vi "Read State DVR.vi"(8 "error in (no error)":errorcluster, 11 "Check Ozone Stability in":refnum<class "Check Ozone Stability.lvclass">) -> (0 "error out":errorcluster, 2 "State DVR":refnum<data-value>, 3 "Check Ozone Stability out":refnum<class "Check Ozone Stability.lvclass">)   [LabVIEW 2013, in "Check Ozone Stability.lvclass"]
uses:
  Check Ozone Stability.lvclass
  Data/cPAS Data.lvclass
  Check Ozone Stability.lvclass/Check Ozone Stability.ctl
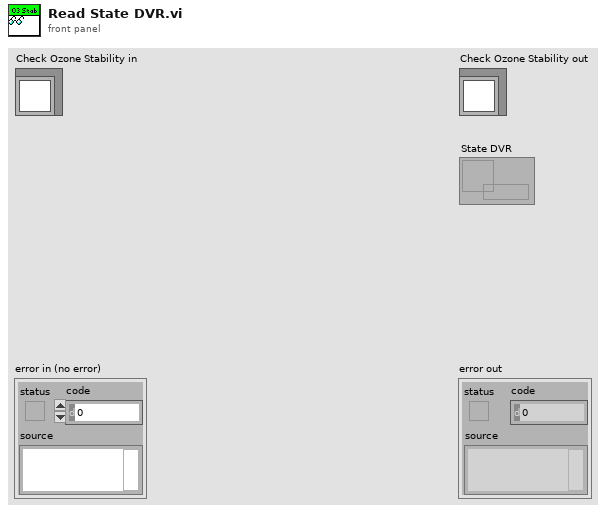
[diagram p1: front panel]
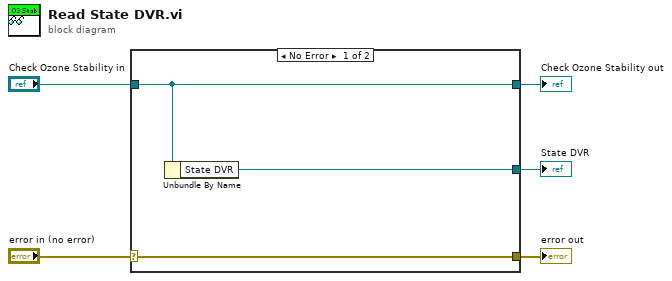
[diagram p0: block diagram]
diagram:
  n1 = case shown="No Error" "error in (no error)" {
    selector: "error in (no error)" -> [w8 w9]
    tunnel: [w8 w9] -> w4
    tunnel: [w7 w10] -> w2
    tunnel: "Check Ozone Stability in" -> [w7 w10]
    tunnel: [w6 _] -> w1
    frame No Error {
      n2 = Unbundle By Name(w7) -> ("State DVR"=w6:refnum<data-value>)
    }
    frame Error {
    }
  }
  "error out" <- w4
  "Check Ozone Stability out" <- w2
  "State DVR" <- w1
